vi "A33ConfigureARB_bk.vi"(0 "VISA resource name":refnum<visa-resource-name>, 1 "ARB Number":i16=1, 2 "Filter (0: OFF)":u16(ring) items=["OFF", "STEP", "NORM"], 3 "Advance mode (0: norm; 1:trig)":u16(ring) items=["Normal", "Triggered"], 5 "Channel (1: Channel1)":u16(ring)=1 items=["Channel1"=1, "Channel2"=2], 7 "Phase (0 deg)":dbl format="%#_12g", 9 "Amplitude (1.0 Vpp)":dbl=1.0 format="%#_12g", 11 "error in (no error)":errorcluster, 12 "DC Offset (0.0 V)":dbl format="%#_12g", 13 "F/SR/P? (0: Frequency)":u16(ring) items=["Frequency", "Sample rate", "Period"], 14 "Freq/SRate/Period (1 Hz)":dbl=1.0 format="%#_12g") -> (4 "VISA resource name out":refnum<visa-resource-name>, 15 "error out":errorcluster)   [LabVIEW 2015]
doc: "Selects the waveform shape, frequency, amplitude, offset, and phase for a standard waveform."
panel:
  # "Positive # - selects wfm from volatile. Wfm must be loaded first.\nNegative - selects wfm loaded from non-vol memory, wfm must be first loaded into volatile from file!"
  # "Sometimes shows error message - it's ok, it's just\nphase sync command"
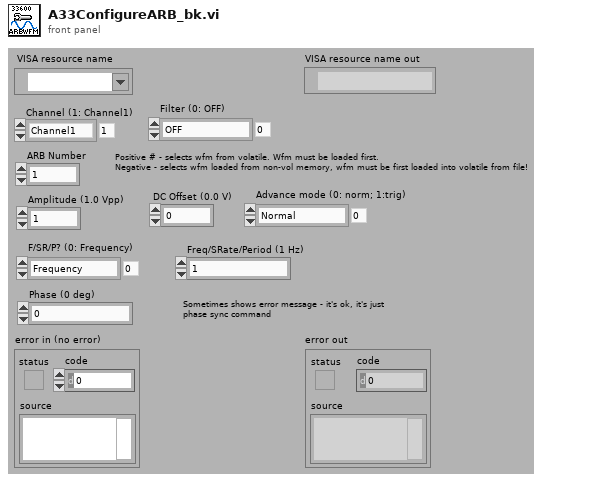
[diagram p1: front panel]
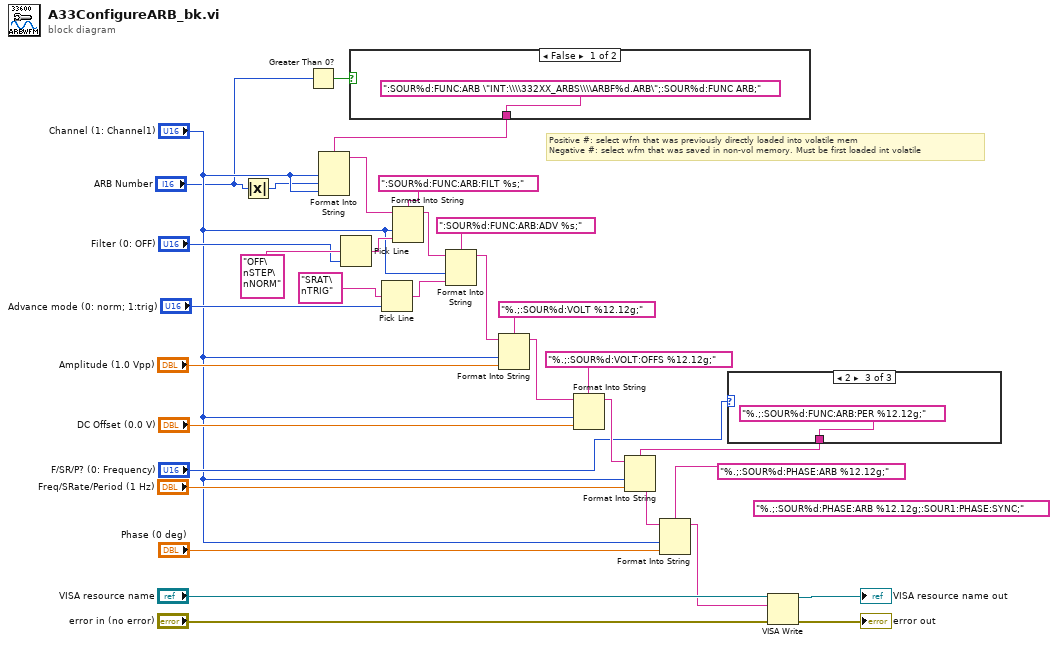
[diagram p0: block diagram]
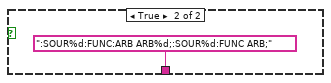
[diagram p2: hidden frame]
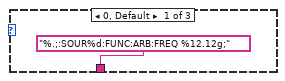
[diagram p3: hidden frame]
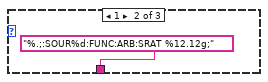
[diagram p4: hidden frame]
diagram:
  (unwired) "%.;:SOUR%d:PHASE:ARB %12.12g;:SOUR1:PHASE:SYNC;"
  # "Positive #: select wfm that was previously directly loaded into volatile mem\nNegative #: select wfm that was saved in non-vol memory. Must be first loaded int volatile"
  n1 = Absolute Value(x="ARB Number") -> (abs(x)=w3:i16)
  n2 = Greater Than 0?(x="ARB Number") -> (x > 0?=w5:bool)
  n3 = Pick Line(multi-line string="OFF\nSTEP\nNORM", line index="Filter (0: OFF)") -> (output string=w17:string)  [unwired: 1 in]
  n4 = case shown="False" w5 {
    tunnel: [":SOUR%d:FUNC:ARB \"INT:\\\\332XX_ARBS\\\\ARBF%d.ARB\";:SOUR%d:FUNC ARB;" ":SOUR%d:FUNC:ARB ARB%d;:SOUR%d:FUNC ARB;"] -> w33
    frame False {
    }
    frame True {
    }
  }
  n5 = Format Into String(format string=w33, "Channel (1: Channel1)", w3, "Channel (1: Channel1)") -> (resulting string=w7:string)  [unwired: 2 in, 1 out]
  n6 = Pick Line(multi-line string="SRAT\nTRIG", line index="Advance mode (0: norm; 1:trig)") -> (output string=w13:string)  [unwired: 1 in]
  n7 = Format Into String(format string=":SOUR%d:FUNC:ARB:FILT %s;" ("string"), initial string=w7, "Channel (1: Channel1)", w17) -> (resulting string=w6:string)  [unwired: 1 in, 1 out]
  n8 = Format Into String(format string=":SOUR%d:FUNC:ARB:ADV %s;", initial string=w6, "Channel (1: Channel1)", w13) -> (resulting string=w14:string)  [unwired: 1 in, 1 out]
  n9 = Format Into String(format string="%.;:SOUR%d:VOLT %12.12g;", initial string=w14, "Channel (1: Channel1)", "Amplitude (1.0 Vpp)") -> (resulting string=w9:string)  [unwired: 1 in, 1 out]
  n10 = Format Into String(format string="%.;:SOUR%d:VOLT:OFFS %12.12g;", initial string=w9, "Channel (1: Channel1)", "DC Offset (0.0 V)") -> (resulting string=w28:string)  [unwired: 1 in, 1 out]
  n11 = case shown="2" "F/SR/P? (0: Frequency)" {
    tunnel: ["%.;:SOUR%d:FUNC:ARB:FREQ %12.12g;" "%.;:SOUR%d:FUNC:ARB:SRAT %12.12g;" "%.;:SOUR%d:FUNC:ARB:PER %12.12g;"] -> w22
    frame 0, Default {
    }
    frame 1 {
    }
    frame 2 {
    }
  }
  n12 = Format Into String(format string=w22, initial string=w28, "Channel (1: Channel1)", "Freq/SRate/Period (1 Hz)") -> (resulting string=w2:string)  [unwired: 1 in, 1 out]
  n13 = Format Into String(format string="%.;:SOUR%d:PHASE:ARB %12.12g;", initial string=w2, "Channel (1: Channel1)", "Phase (0 deg)") -> (resulting string=w1:string)  [unwired: 1 in, 1 out]
  n14 = VISA Write(VISA resource name="VISA resource name", write buffer=w1, error in (no error)="error in (no error)") -> (VISA resource name out=→"VISA resource name out":refnum<visa-resource-name>, error out=→"error out":errorcluster)  [unwired: 1 out]
